vi "TEST loop timing.vi"() -> ()   [LabVIEW 2023]
uses:
  <vilib>/Rock Robotics/WPI/ThirdParty/JAS_Junk/TrajLib/TypeDef/TIMER.ctl
  <vilib>/Utility/semaphor.llb/Obtain Semaphore Reference.vi
  <vilib>/Rock Robotics/WPI/ThirdParty/JAS_Junk/TrajLib/Timer_Reset.vi
  <vilib>/Rock Robotics/WPI/ThirdParty/JAS_Junk/TrajLib/Trajectory_Library.lvlib
panel:
  out "CurrentTImer":dbl
  in  "TIMER":T1 {"Accumulated TIme" format="%13.5p"; "StartTime" format="%13.5p"}
  in  "loop (s)":dbl
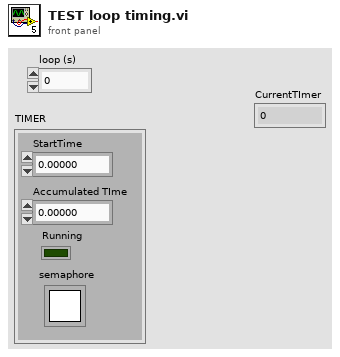
[diagram p1: front panel]
types:
  T1 = typedef "Trajectory_Library.lvlib/TIMER.ctl" = cluster{"StartTime":dbl, "Accumulated TIme":dbl, "Running":bool, "semaphore":T2}
  T2 = typedef "Semaphore RefNum" = refnum<k1>
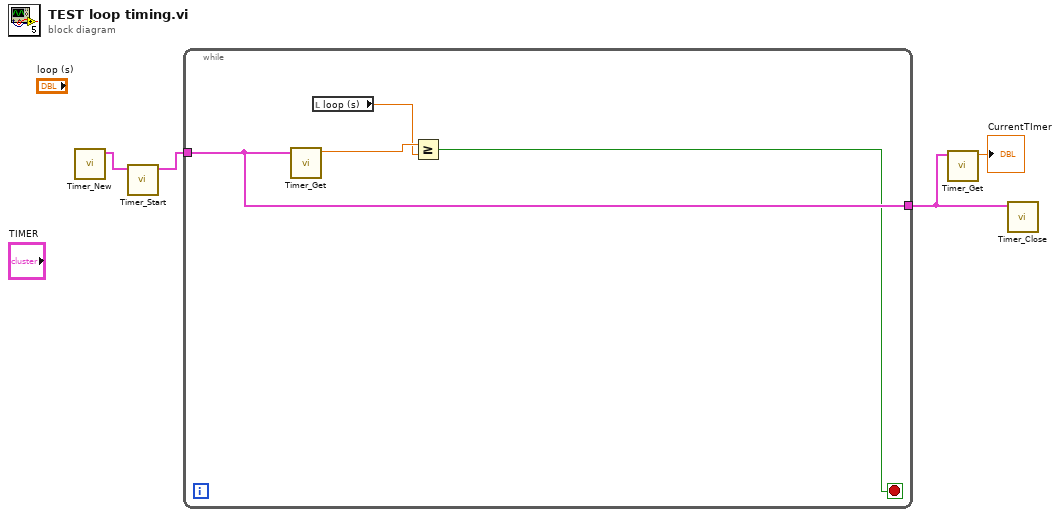
[diagram p0: block diagram]
diagram:
  n1 = call <vilib>:"Timer_New.vi"() -> ("TIMER"=w1:T1)  [unwired: 11 in]
  n2 = call <vilib>:"Timer_Start.vi"("in Timer"=w1) -> ("out Timer"=w2:T1)  [unwired: 10 in]
  n3 = while {
    tunnel: w2 -> [w8]
    tunnel: [w8] -> w4
    stop <- w5 stop-if-true
    n4 = call <vilib>:"Timer_Get.vi"("TIMER"=w8) -> ("CurrentTImer"=w7:dbl)  [unwired: 10 in]
    n5 = local read "loop (s)"() -> (w6:dbl)
    n6 = Greater Or Equal?(x=w7, y=w6) -> (x >= y?=w5:bool)
  }
  n7 = call <vilib>:"Timer_Get.vi"("TIMER"=w4) -> ("CurrentTImer"=→"CurrentTImer":dbl)  [unwired: 10 in]
  n8 = call <vilib>:"Timer_Close.vi"("TIMER"=w4) -> ()  [unwired: 11 in]
